vi "Write_Diagnostics_Used_to_String.vi"(1 "| B-dot 2 |":bool=TRUE, 2 "| B-dot 1 |":bool=TRUE, 3 "| Rogowski 3 |":bool=TRUE, 4 "| Rogowski 2 |":bool=TRUE, 5 "| Rogowski 1 |":bool=TRUE, 6 "| Lanmuir Probe |":bool=TRUE) -> (0 "String":string)   [LabVIEW 2017]
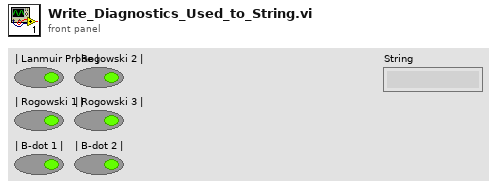
[diagram p1: front panel]
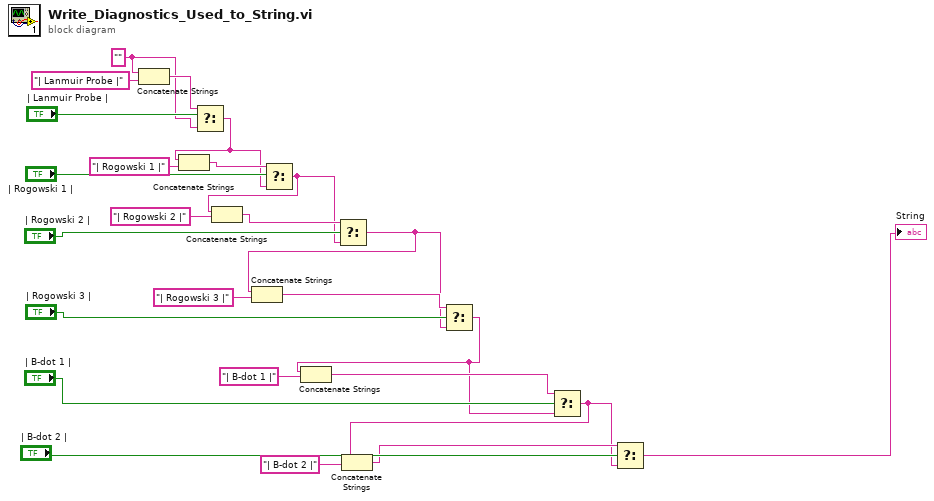
[diagram p0: block diagram]
diagram:
  w22 = ""
  n1 = Concatenate Strings(w22, "| Lanmuir Probe |" ("string")) -> (w24:string)
  n2 = Select(t=w24, s="| Lanmuir Probe |", f=w22) -> (s? t:f=w14:string)
  n3 = Concatenate Strings(w14, "| Rogowski 1 |" ("string")) -> (w15:string)
  n4 = Select(t=w15, s="| Rogowski 1 |", f=w14) -> (s? t:f=w7:string)
  n5 = Concatenate Strings(w7, "| Rogowski 2 |" ("string")) -> (w8:string)
  n6 = Select(t=w8, s="| Rogowski 2 |", f=w7) -> (s? t:f=w5:string)
  n7 = Concatenate Strings(w5, "| Rogowski 3 |" ("string")) -> (w6:string)
  n8 = Select(t=w6, s="| Rogowski 3 |", f=w5) -> (s? t:f=w3:string)
  n9 = Concatenate Strings(w3, "| B-dot 1 |" ("string")) -> (w4:string)
  n10 = Select(t=w4, s="| B-dot 1 |", f=w3) -> (s? t:f=w1:string)
  n11 = Concatenate Strings(w1, "| B-dot 2 |" ("string")) -> (w2:string)
  n12 = Select(t=w2, s="| B-dot 2 |", f=w1) -> (s? t:f=→"String":string)
